vi "DilutionVisible.vi"(0 "calculated":u16) -> (1 "flow":u16(ring)=2 items=["Enabled", "Disabled", "Disabled and Grayed Out"], 2 "MFC1":u16(ring)=2 items=["Enabled", "Disabled", "Disabled and Grayed Out"], 3 "MFC2":u16(ring)=2 items=["Enabled", "Disabled", "Disabled and Grayed Out"], 4 "MFC3":u16(ring)=2 items=["Enabled", "Disabled", "Disabled and Grayed Out"])   [LabVIEW 2011]
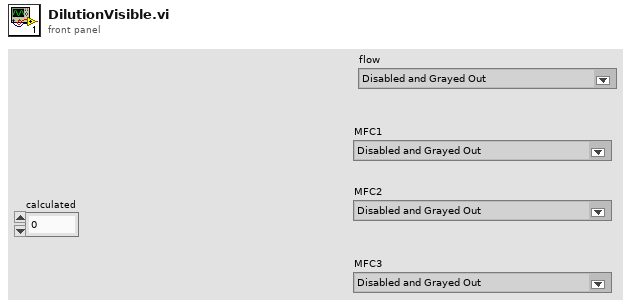
[diagram p1: front panel]
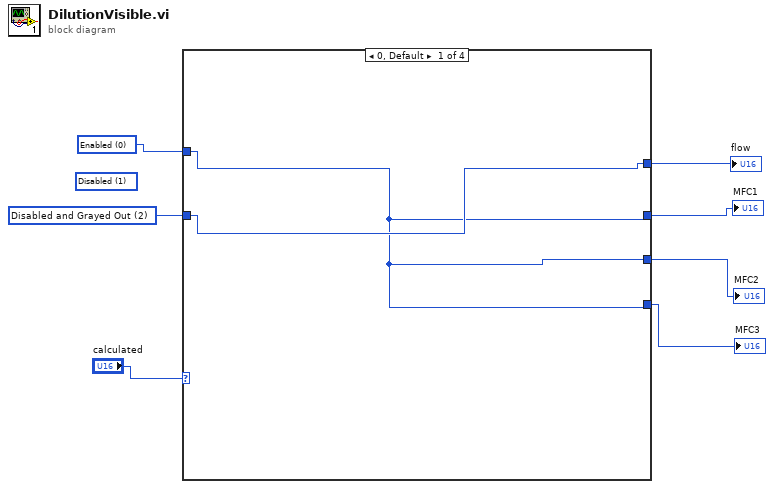
[diagram p0: block diagram]
diagram:
  w4 = u16 2 items=["Enabled", "Disabled", "Disabled and Grayed Out"] ("flow 2")
  (unwired) u16 1 items=["Enabled", "Disabled", "Disabled and Grayed Out"] ("flow 2")
  w5 = u16 0 items=["Enabled", "Disabled", "Disabled and Grayed Out"] ("flow 2")
  n1 = case shown="0, Default" "calculated" {
    tunnel: [w9 w11 w13 w15] -> w6
    tunnel: w5 -> [w8 w11 w13 w15]
    tunnel: w4 -> [w9 w10 w12 w14]
    tunnel: [w8 w11 w13 w14] -> w3
    tunnel: [w8 w10 w13 w15] -> w2
    tunnel: [w8 w11 w12 w15] -> w1
    frame 0, Default {
    }
    frame 1 {
    }
    frame 2 {
    }
    frame 3 {
    }
  }
  "flow" <- w6
  "MFC1" <- w2
  "MFC2" <- w1
  "MFC3" <- w3
